vi "ClimbLogic.vi"() -> ()   [LabVIEW 2018]
uses:
  <vilib>/Rock Robotics/WPI/ThirdParty/Phoenix-LabVIEW/Motor Controller/Controls/CTRE_Phoenix_MotorControl_ControlMode.ctl
  <vilib>/Rock Robotics/WPI/Relay/WPI_RelayValue.ctl
  <vilib>/Rock Robotics/WPI/Utilities/WPI_GetSetVariantRefNum.vi
  Globals.vi
  <vilib>/Rock Robotics/WPI/ThirdParty/Phoenix-LabVIEW/Motor Controller/Get/CTRE_Phoenix_MotorController_GetLimitSwitchStates.vi
  <vilib>/Rock Robotics/Network Tables/NT Write Numeric Array.vi
panel:
  in  "ClimbLevel":enum16{"2", "3"}(ring)
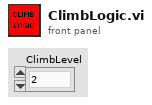
[diagram p1: front panel]
types:
  T1 = typedef "WPI_AnalogChannelDevRef.ctl" = cluster{"DevStatus":errorcluster, "Analog Channel":T2}
  T2 = typedef "FPGA_AIChannel.ctl" = enum8{"AI 0", "AI 1", "AI 2", "AI 3", "AI MXP 0", "AI MXP 1", "AI MXP 2", "AI MXP 3", "Invalid"}
  T3 = typedef "WPI_RelayDevRef.ctl" = cluster{"DevStatus":errorcluster, "Relay Channel":T4, "Relay Direction":T5}
  T4 = typedef "FPGA_DIORelayChannel.ctl" = enum8{"Relay 0", "Relay 1", "Relay 2", "Relay 3", "Invalid"}
  T5 = typedef "WPI_RelayDirection.ctl" = enum16{"Both directions", "Forward only", "Reverse only"}
  T6 = typedef "WPI_JoystickDevRef.ctl" = cluster{"Device":T7}
  T7 = typedef "WPI_JoystickDeviceEnum.ctl" = enum16{"USB 0", "USB 1", "USB 2", "USB 3", "USB 4", "USB 5"}
  T8 = typedef "WPI_MotorControlDeviceRef.ctl" = cluster{"DeviceStatus":errorcluster, "Type":T9, "PWM":cluster{"PWM Channel":T10, "DeadBand":T11}, "CAN":cluster{"Device Number":u8, "SetOutput VI Ref":variant, "GetOutput VI Ref":variant, "Enable VI Ref":variant, "Disable VI Ref":variant, "Data":variant}, "Invert":bool, "DIO PWM":cluster{"PWM \"Enable\" Channel":T10, "DIOChannel":T12, "PWM Rate":dbl}}
  T9 = typedef "WPI_MotorControlType.ctl" = enum16{"PWM", "CAN", "DIO PWM"}
  T10 = typedef "FPGA_DIOPWMChannel.ctl" = enum8{"PWM 0", "PWM 1", "PWM 2", "PWM 3", "PWM 4", "PWM 5", "PWM 6", "PWM 7", "PWM 8", "PWM 9", "PWM MXP 0", "PWM MXP 1", "PWM MXP 2", "PWM MXP 3", "PWM MXP 4", "PWM MXP 5", "PWM MXP 6", "PWM MXP 7", "PWM MXP 8", "PWM MXP 9", "Invalid"}
  T11 = typedef "WPI_PWMDeadband.ctl" = cluster{"Name":string, "maxPositivePwm":i32, "minPositivePwm":i32, "centerPwm":i32, "maxNegativePwm":i32, "minNegativePwm":i32, "angularRange":u16}
  T12 = typedef "FPGA_DIOChannel.ctl" = enum8{"DIO 0", "DIO 1", "DIO 2", "DIO 3", "DIO 4", "DIO 5", "DIO 6", "DIO 7", "DIO 8", "DIO 9", "DIO MXP 0", "DIO MXP 1", "DIO MXP 2", "DIO MXP 3", "DIO MXP 4", "DIO MXP 5", "DIO MXP 6", "DIO MXP 7", "DIO MXP 8", "DIO MXP 9", "DIO MXP 10", "DIO MXP 11", "DIO MXP 12", "DIO MXP 13", "DIO MXP 14", "DIO MXP 15", "SPI Port CS1", "SPI Port CS2", "SPI Port CS3", "SPI Port MISO", "SPI Port MOSI", "Invalid"}
  T13 = typedef "WPI_EncoderDevRef.ctl" = cluster{"DevStatus":errorcluster, "EncoderIndex":T14, "CounterIndex":T15, "DistancePerCount":dbl, "Decoding Type":T16}
  T14 = typedef "FPGA_EncoderIdx.ctl" = enum8{"Enc 0", "Enc 1", "Enc 2", "Enc 3", "Enc 4", "Enc 5", "Enc 6", "Enc 7", "Invalid"}
  T15 = typedef "FPGA_CounterCtrSystemIndex.ctl" = enum8{"Ctr 0", "Ctr 1", "Ctr 2", "Ctr 3", "Ctr 4", "Ctr 5", "Ctr 6", "Ctr 7", "Invalid"}
  T16 = typedef "WPI_EncoderType.ctl" = enum16{"1x", "2x", "4x"}
  T17 = typedef "WPI_RelayValue.ctl" = enum16{"Off", "On", "Forward", "Reverse"}
  T18 = enum16{"initial climb", "elevated drive", "retract 1", "on platform drive", "retract 2", "finish"}
  T19 = typedef "CTRE_Phoenix_MotorControl_ControlMode.ctl" = u16
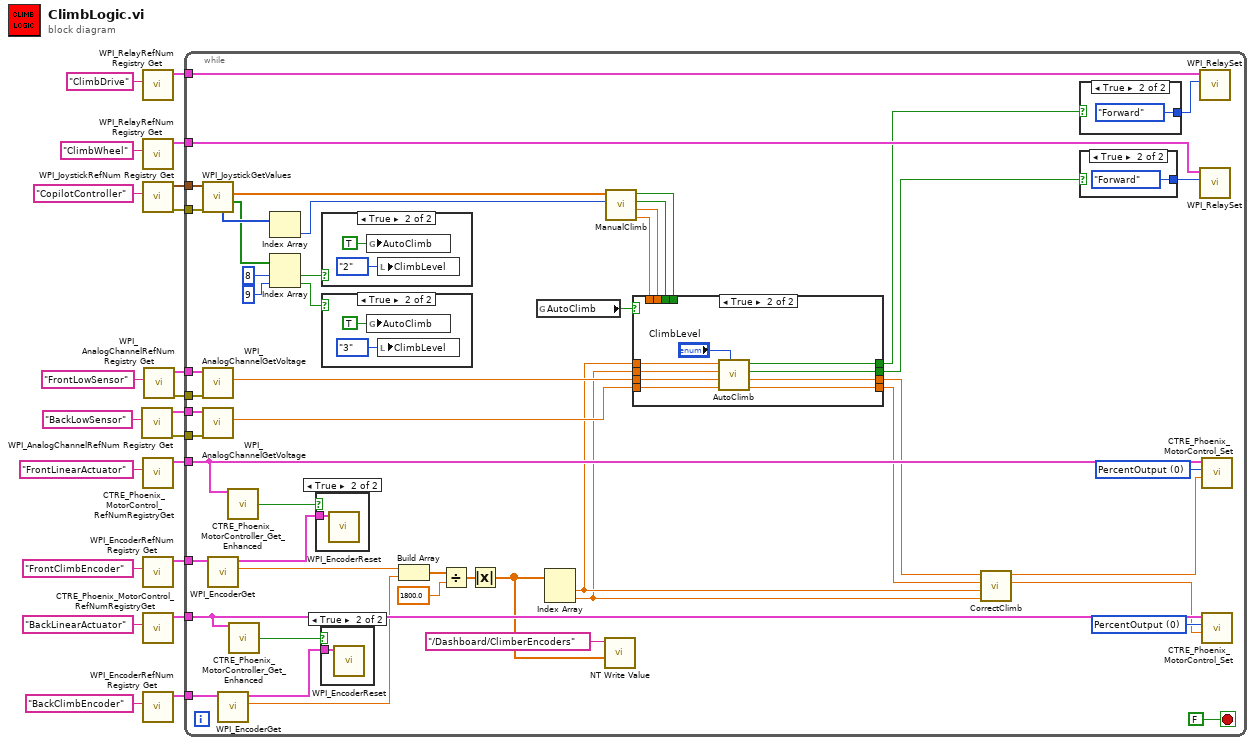
[diagram p0: block diagram]
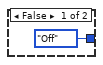
[diagram p4: hidden frame]
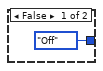
[diagram p7: hidden frame]
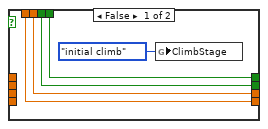
[diagram p8: hidden frame]
diagram:
  n1 = call <vilib>:"WPI_AnalogChannelRefNum Registry Get.vi"("refnum name"="BackLowSensor") -> ("error out"=w1:errorcluster, "AIDeviceRef"=w9:T1)  [unwired: 9 in]
  n2 = call <vilib>:"WPI_RelayRefNum Registry Get.vi"("refnum name"="ClimbDrive") -> ("RelayDevRef"=w11:T3)  [unwired: 9 in, 1 out]
  n3 = call <vilib>:"WPI_RelayRefNum Registry Get.vi"("refnum name"="ClimbWheel") -> ("RelayDevRef"=w8:T3)  [unwired: 9 in, 1 out]
  n4 = call <vilib>:"WPI_JoystickRefNum Registry Get.vi"("refnum name"="CopilotController") -> ("error out"=w3:errorcluster, "JoystickDevRef"=w12:T6)  [unwired: 1 in, 8 out]
  n5 = call <vilib>:"CTRE_Phoenix_MotorControl_RefNumRegistryGet.vi"("refnum name"="FrontLinearActuator") -> ("PhoenixMotorControlDevRef"=w7:T8)  [unwired: 9 in, 1 out]
  n6 = call <vilib>:"WPI_EncoderRefNum Registry Get.vi"("refnum name"="FrontClimbEncoder") -> ("EncoderDevRef"=w6:T13)  [unwired: 9 in, 1 out]
  n7 = call <vilib>:"CTRE_Phoenix_MotorControl_RefNumRegistryGet.vi"("refnum name"="BackLinearActuator") -> ("PhoenixMotorControlDevRef"=w5:T8)  [unwired: 9 in, 1 out]
  n8 = call <vilib>:"WPI_EncoderRefNum Registry Get.vi"("refnum name"="BackClimbEncoder") -> ("EncoderDevRef"=w4:T13)  [unwired: 9 in, 1 out]
  n9 = call <vilib>:"WPI_AnalogChannelRefNum Registry Get.vi"("refnum name"="FrontLowSensor") -> ("error out"=w2:errorcluster, "AIDeviceRef"=w10:T1)  [unwired: 9 in]
  n10 = while {
    tunnel: w12 -> [w65]
    tunnel: w11 -> [w30]
    tunnel: w10 -> [w64]
    tunnel: w9 -> [w63]
    tunnel: w8 -> [w62]
    tunnel: w7 -> [w61]
    tunnel: w6 -> [w60]
    tunnel: w5 -> [w59]
    tunnel: w4 -> [w58]
    tunnel: w3 -> [w57]
    tunnel: w2 -> [w37]
    tunnel: w1 -> [w36]
    stop <- FALSE stop-if-true
    w46 = T19 0 items=["PercentOutput"=0, "Position"=1, "Velocity"=2, "Current"=3, "Follower"=5, "MotionProfile"=6, "MotionMagic"=7, "MotionProfileArc"=10, "Disabled"=15] ("Control Mode")
    w47 = T19 0 items=["PercentOutput"=0, "Position"=1, "Velocity"=2, "Current"=3, "Follower"=5, "MotionProfile"=6, "MotionMagic"=7, "MotionProfileArc"=10, "Disabled"=15] ("Control Mode")
    n11 = call <vilib>:"WPI_JoystickGetValues.vi"("error in (no error)"=w57, "JoystickDevRef"=w65) -> ("Buttons"=w54:bool[], "Axes"=w72:dbl[], "POVs"=w56:i16[])  [unwired: 5 in, 2 out]
    n12 = call <vilib>:"WPI_AnalogChannelGetVoltage.vi"("error in (no error)"=w37, "AIDeviceRef"=w64) -> ("Voltage"=w70:dbl)  [unwired: 7 in, 2 out]
    n13 = call <vilib>:"WPI_AnalogChannelGetVoltage.vi"("error in (no error)"=w36, "AIDeviceRef"=w63) -> ("Voltage"=w71:dbl)  [unwired: 7 in, 2 out]
    n14 = call <vilib>:"WPI_EncoderGet.vi"("EncoderDevRef"=w60) -> ("Distance"=w43:dbl, "EncoderDevRef"=w67:T13)  [unwired: 5 in, 4 out]
    n15 = call <vilib>:"WPI_EncoderGet.vi"("EncoderDevRef"=w58) -> ("Distance"=w44:dbl, "EncoderDevRef"=w68:T13)  [unwired: 5 in, 4 out]
    n16 = call-poly <vilib>:"CTRE_Phoenix_MotorController_Get_Enhanced.vi"("PhoenixMotorControlDevRef"=w61) -> ("Reverse Limit Closed?"=w49:bool)  [unwired: 11 in, 3 out]
    n17 = call-poly <vilib>:"CTRE_Phoenix_MotorController_Get_Enhanced.vi"("PhoenixMotorControlDevRef"=w59) -> ("Reverse Limit Closed?"=w48:bool)  [unwired: 11 in, 3 out]
    n18 = Index Array(array=w56) -> (element=w55:i16)  [unwired: 1 in]
    n19 = Index Array(array=w54, index #1=8 ("index"), index #2=9 ("index")) -> (element #1=w53:bool, element #2=w51:bool)
    n20 = case shown="True" w49 {
      tunnel: w67 -> [_ w80]
      frame False {
      }
      frame True {
        n21 = call <vilib>:"WPI_EncoderReset.vi"("EncoderDevRef"=w80) -> ()  [unwired: 9 in, 2 out]
      }
    }
    n22 = case shown="True" w48 {
      tunnel: w68 -> [_ w79]
      frame False {
      }
      frame True {
        n23 = call <vilib>:"WPI_EncoderReset.vi"("EncoderDevRef"=w79) -> ()  [unwired: 9 in, 2 out]
      }
    }
    n24 = case shown="True" w53 {
      frame False {
      }
      frame True {
        n25 = global write "Globals.vi" "AutoClimb"(TRUE ("AutoClimb")) -> ()
        n26 = local write "ClimbLevel"(enum16{"2", "3"}."2" ("ClimbLevel")) -> ()
      }
    }
    n27 = case shown="True" w51 {
      frame False {
      }
      frame True {
        n28 = global write "Globals.vi" "AutoClimb"(TRUE ("AutoClimb")) -> ()
        n29 = local write "ClimbLevel"(enum16{"2", "3"}."3" ("ClimbLevel")) -> ()
      }
    }
    n30 = Build Array(w43, w44) -> (w32:dbl[])
    n31 = Divide(x=w32, y=1800.0) -> (x/y=w45:dbl[])
    n32 = Absolute Value(x=w45) -> (abs(x)=w28:dbl[])
    n33 = global read "Globals.vi" "AutoClimb"() -> (w35:bool)
    n34 = Index Array(array=w28) -> (element #1=w26:dbl, element #2=w22:dbl)  [unwired: 2 in]
    n35 = call-poly <vilib>:"NT Write Value.vi"("Numeric Array"=w28, "Name"="/Dashboard/ClimberEncoders") -> ()  [unwired: 9 in, 1 out]
    n36 = call "ManualClimb.vi"("CopilotPOV"=w55, "CopilotAxes"=w72) -> ("ActuateBackClimb"=w40:dbl, "ActuateFrontClimb"=w34:dbl, "DropWheel"=w41:bool, "ClimbDrive"=w42:bool)  [unwired: 6 in]
    n37 = case shown="True" w35 {
      tunnel: w26 -> [_ w96]
      tunnel: w22 -> [_ w93]
      tunnel: w70 -> [_ w95]
      tunnel: w71 -> [_ w94]
      tunnel: [w87 w91] -> w39
      tunnel: w42 -> [w87 _]
      tunnel: [w86 w90] -> w33
      tunnel: w41 -> [w86 _]
      tunnel: [w85 w88] -> w23
      tunnel: w34 -> [w85 _]
      tunnel: [w84 w89] -> w27
      tunnel: w40 -> [w84 _]
      frame False {
        n38 = global write "Globals.vi" "ClimbStage"(T18."initial climb" ("ClimbStage")) -> ()
      }
      frame True {
        n39 = call "AutoClimb.vi"("ClimbLevel"="ClimbLevel", "BackLowSensor"=w94, "FrontLowSensor"=w95, "BackClimbEncoder"=w93, "FrontClimbEncoder"=w96) -> ("ActuateBackClimb"=w89:dbl, "ActuateFrontClimb"=w88:dbl, "DropWheel"=w90:bool, "ClimbDrive"=w91:bool)  [unwired: 3 in]
      }
    }
    n40 = call "CorrectClimb.vi"("BackEncoder"=w22, "FrontEncoder"=w26, "BackControl"=w27, "FrontControl"=w23) -> ("BackOutput"=w24:dbl, "FrontOutput"=w25:dbl)  [unwired: 6 in]
    n41 = case shown="True" w39 {
      tunnel: [WPI_RelayValue."Off" ("RelayValue") WPI_RelayValue."Forward" ("RelayValue")] -> w66
      frame False {
      }
      frame True {
      }
    }
    n42 = case shown="True" w33 {
      tunnel: [WPI_RelayValue."Off" ("RelayValue") WPI_RelayValue."Forward" ("RelayValue")] -> w69
      frame False {
      }
      frame True {
      }
    }
    n43 = call <vilib>:"WPI_RelaySet.vi"("RelayValue"=w66, "RelayDevRef"=w30) -> ()  [unwired: 8 in, 2 out]
    n44 = call <vilib>:"WPI_RelaySet.vi"("RelayValue"=w69, "RelayDevRef"=w62) -> ()  [unwired: 8 in, 2 out]
    n45 = call <vilib>:"CTRE_Phoenix_MotorControl_Set.vi"("Output"=w25, "Control Mode"=w47, "PhoenixMotorControlDevRef"=w61) -> ()  [unwired: 7 in, 2 out]
    n46 = call <vilib>:"CTRE_Phoenix_MotorControl_Set.vi"("Output"=w24, "Control Mode"=w46, "PhoenixMotorControlDevRef"=w59) -> ()  [unwired: 7 in, 2 out]
  }
